vi "Reload Configuration.vi"(8 "error in (no error)":errorcluster, 11 "Cfg Grandmaster in":refnum<class "Cfg Grandmaster.lvclass">) -> (0 "error out":errorcluster, 3 "Cfg Grandmaster out":refnum<class "Cfg Grandmaster.lvclass">)   [LabVIEW 2018, in "Configuration Grandmaster.lvlib" / "Cfg Grandmaster.lvclass"]
uses:
  Cfg Grandmaster.lvclass
  Cfg Grandmaster.lvclass/Cfg Grandmaster.ctl
  Class Chassis BOM/Chassis BOM.lvclass/Chassis BOM.ctl
  Class Chassis BOM/Read CfgFile.vi
  Class FP Ctrls/FP Controls.lvclass
  Class Chassis BOM/Chassis BOM.lvclass
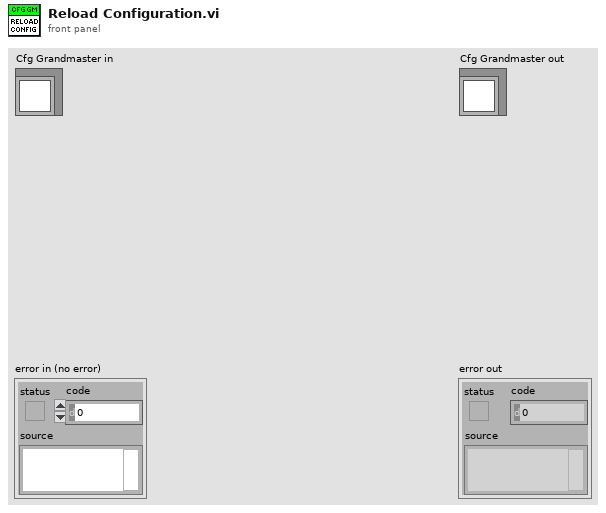
[diagram p1: front panel]
types:
  T1 = typedef "ge_Cfg wChassis.ctl" = cluster{"Chassis BOM":refnum<class "Chassis BOM.lvclass">, "Chassis Cfg":refnum<class "ChassisCfg.lvclass">, "Chassis Tasks":refnum<class "Chassis Tasks.lvclass">, "HW Error":bool, "Unsvd Chgs?":bool}
  T2 = typedef "Selected Group.ctl" = cluster{"ChanGroup":i32, "Rate Class":T3}
  T3 = typedef "TE_Designator.ctl" = enum16{"High Speed", "Low Speed"}
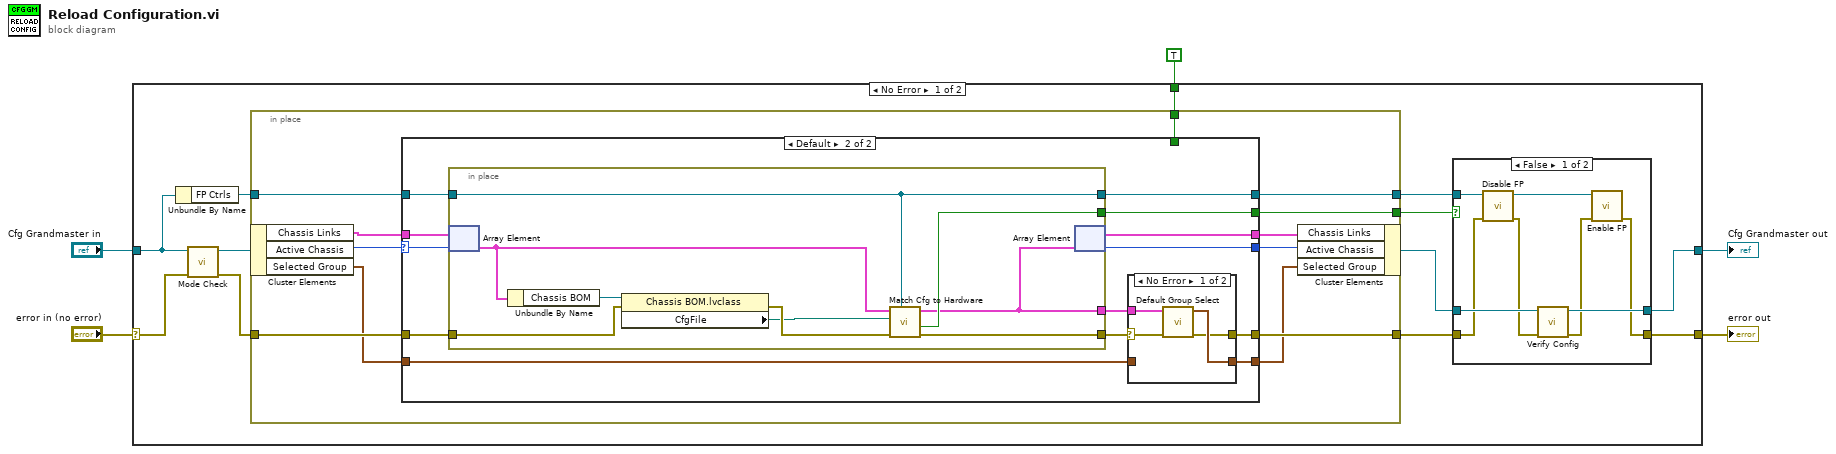
[diagram p0: block diagram]
diagram:
  n1 = case shown="No Error" "error in (no error)" {
    selector: "error in (no error)" -> [w15 w75]
    tunnel: [w6 w75] -> w4
    tunnel: [w13 w74] -> w2
    tunnel: "Cfg Grandmaster in" -> [w10 w74]
    tunnel: TRUE ("HW Error?") -> [w17 _]
    frame No Error {
      n2 = Unbundle By Name(w10) -> ("FP Ctrls"=w9:refnum<class "FP Controls.lvclass">)
      n3 = call "Mode Check.vi"("error in (no error)"=w15, "Cfg Grandmaster in"=w10) -> ("error out"=w8:errorcluster, "Cfg Grandmaster out"=w16:refnum<class "Cfg Grandmaster.lvclass">)  [unwired: 8 in]
      n4 = in-place {
        in-place-border: w8 -> [w39]
        in-place-border: [w38] -> w14
        in-place-border: [w35] -> w11
        in-place-border: w17 -> [w30]
        in-place-border: w9 -> [w29]
        in-place-border: [w28] -> w7
        n5 = in-place-cluster #1(w16) -> ("Chassis Links"=w37:T1[], "Active Chassis"=w32:i32, "Selected Group"=w34:T2)
        n6 = case shown="Default" w32 {
          selector: w32 -> [w42 w52]
          tunnel: [w44 w54] -> w38
          tunnel: [w45 w51] -> w36
          tunnel: w34 -> [w43 w49]
          tunnel: w37 -> [w45 w53]
          tunnel: [w41 w58] -> w35
          tunnel: w39 -> [w44 w57]
          tunnel: [w43 w55] -> w33
          tunnel: [w42 w48] -> w31
          tunnel: w30 -> [w41 _]
          tunnel: w29 -> [w40 w47]
          tunnel: [w40 w46] -> w28
          frame -1 {
          }
          frame Default {
            n7 = in-place {
              in-place-border: [w73] -> w58
              in-place-border: w57 -> [w70]
              in-place-border: [w71] -> w56
              in-place-border: [w72] -> w50
              in-place-border: w47 -> [w65]
              in-place-border: [w65] -> w46
              n8 = in-place-array #2(w53, w52) -> (w67:T1)
              n9 = Unbundle By Name(w67) -> ("Chassis BOM"=w68:refnum<class "Chassis BOM.lvclass">)
              n10 = property class="Chassis BOM.lvclass"(reference=w68, error in=w70) -> (error out=w69:errorcluster, "CfgFile"=w66:path)  [unwired: 1 out]
              n11 = call "Match Cfg to Hardware.vi"("FP Ctrls"=w65, "error in"=w69, "selected path"=w66, "Cfg wChassis"=w67) -> ("error out"=w72:errorcluster, "HW Error?"=w73:bool, "Cfg wChassis"=w71:T1)  [unwired: 5 in]
              n12 = in-place-array #2(w71) -> (w51:T1[], w48:i32)
            }
            n13 = case shown="No Error" w50 {
              selector: w50 -> [w59 w63]
              tunnel: w56 -> [w62 _]
              tunnel: [w61 w64] -> w55
              tunnel: [w60 w63] -> w54
              tunnel: w49 -> [_ w64]
              frame No Error {
                n14 = call "Default Group Select.vi"("error in"=w59, "Cfg with Chassis"=w62) -> ("error out"=w60:errorcluster, "Selected Grp"=w61:T2)  [unwired: 8 in]
              }
              frame Error {
              }
            }
          }
        }
        n15 = in-place-cluster #1("Chassis Links"=w36, "Active Chassis"=w31, "Selected Group"=w33) -> (w12:refnum<class "Cfg Grandmaster.lvclass">)
      }
      n16 = case shown="False" w11 {
        tunnel: w14 -> [w21 w26]
        tunnel: [w18 w26] -> w6
        tunnel: [w25 w27] -> w13
        tunnel: w12 -> [w24 w27]
        tunnel: w7 -> [w23 _]
        frame False {
          n17 = call "Disable FP.vi"("error in (no error)"=w21, "FP Controls in"=w23) -> ("error out"=w20:errorcluster, "FP Controls out"=w22:refnum<class "FP Controls.lvclass">)  [unwired: 8 in]
          n18 = call "Verify Config.vi"("error in (no error)"=w20, "Cfg Grandmaster in"=w24) -> ("error out"=w19:errorcluster, "Cfg Grandmaster out"=w25:refnum<class "Cfg Grandmaster.lvclass">)  [unwired: 8 in]
          n19 = call "Enable FP.vi"("error in (no error)"=w19, "FP Controls in"=w22) -> ("error out"=w18:errorcluster)  [unwired: 8 in, 1 out]
        }
        frame True {
        }
      }
    }
    frame Error {
    }
  }
  "error out" <- w4
  "Cfg Grandmaster out" <- w2
